vi "FilePoly.vi"   [LabVIEW 2016]
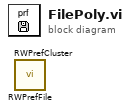
[diagram p0: block diagram]
diagram:
  n1 = call "RWPrefFile.vi"() -> ()  [unwired: 10 in, 2 out]
  n2 = call "RWPrefCluster.vi"() -> ()  [unwired: 10 in, 2 out]
